vi "Properties for Reorder.vi"(11 "Tree Controls":refnum<vi>[](array[refnum])) -> (2 "All Tags":string[](array[string]), 3 "Property Array Out":T1(array[cluster]))   [LabVIEW 2023]
doc: "Output the properties in the new rearranged order."
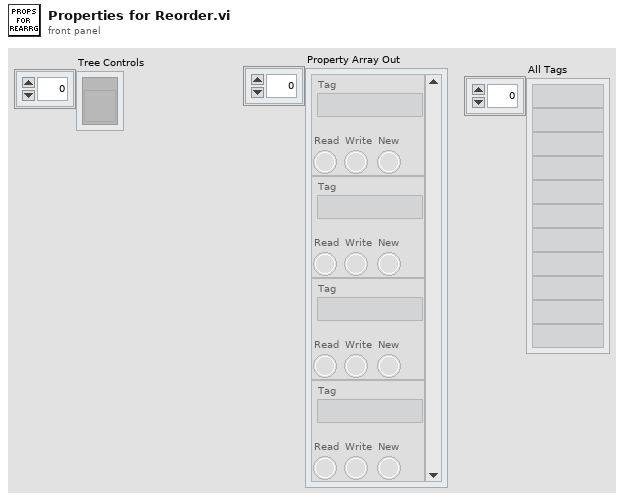
[diagram p1: front panel]
types:
  T1 = cluster{"Tag":string, "Read":bool, "Write":bool, "New":bool}[]
  T2 = cluster{"Tag":string, "Read":bool, "Write":bool, "New":bool}
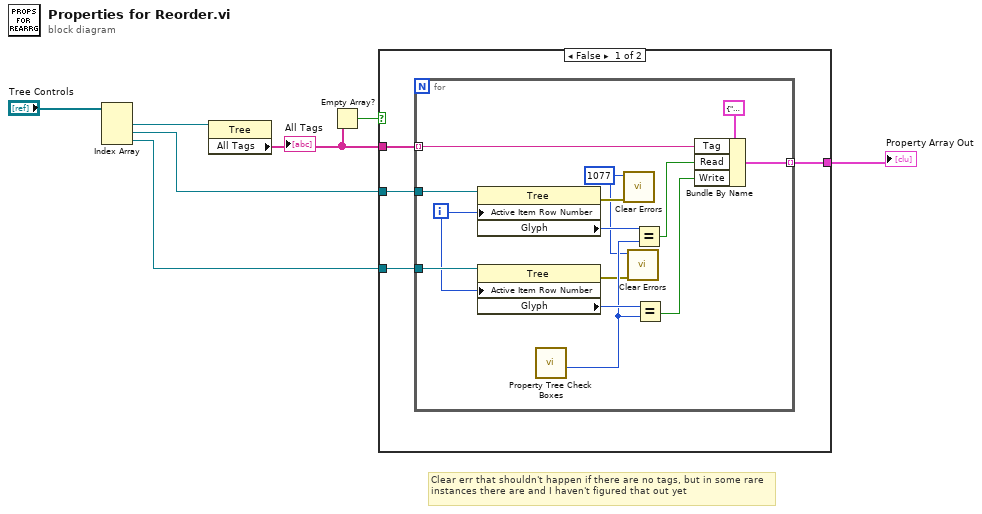
[diagram p0: block diagram]
diagram:
  # "Clear err that shouldn't happen if there are no tags, but in some rare instances there are and I haven't figured that out yet"
  n1 = Index Array(array="Tree Controls") -> (element #1=w6:refnum<vi>, element #2=w5:refnum<vi>, element #3=w4:refnum<vi>)  [unwired: 3 in]
  n2 = property class="Tree"(reference=w6) -> ("All Tags"=w2:string[])  [unwired: 1 in, 2 out]
  "All Tags" <- w2
  n3 = Empty Array?(array=w2) -> (empty?=w1:bool)
  n4 = case shown="False" w1 {
    tunnel: w5 -> [w11 _]
    tunnel: w4 -> [w10 _]
    tunnel: w2 -> [w9 _]
    tunnel: [w8 _] -> w3
    frame False {
      n5 = for {
        tunnel: w11 -> [w25]
        tunnel: w10 -> [w24]
        tunnel: w9 -> [w19] mode=indexing
        tunnel: [w16] -> w8 mode=indexing
        i -> [w15]
        w12 = 1077 ("specific error code to clear (0: all)")
        n6 = property class="Tree"(reference=w25, "Active Item Row Number"=w15) -> (error out=w14:errorcluster, "Glyph"=w23:i32)  [unwired: 1 in, 1 out]
        n7 = property class="Tree"(reference=w24, "Active Item Row Number"=w15) -> (error out=w13:errorcluster, "Glyph"=w22:i32)  [unwired: 1 in, 1 out]
        n8 = call "Property Tree Check Boxes.vi"() -> ("Checked"=w21:i32)  [unwired: 9 in, 2 out]
        n9 = call <vilib>:"Clear Errors.vi"("error in (no error)"=w14, "specific error code to clear (0: all)"=w12) -> ()  [unwired: 4 in, 2 out]
        n10 = call <vilib>:"Clear Errors.vi"("error in (no error)"=w13, "specific error code to clear (0: all)"=w12) -> ()  [unwired: 4 in, 2 out]
        n11 = Equal?(x=w23, y=w21) -> (x = y?=w18:bool)
        n12 = Equal?(x=w22, y=w21) -> (x = y?=w17:bool)
        n13 = Bundle By Name(cluster=T2 {"Tag"="", "Read"=FALSE, "Write"=FALSE, "New"=FALSE} ("Property Tree Element Value"), "Tag"=w19, "Read"=w18, "Write"=w17) -> (w16:T2)
      }
    }
    frame True {
    }
  }
  "Property Array Out" <- w3
